vi "Get or Add Sheets.vi"(8 "error in":errorcluster, 11 "SpreadsheetDoc in":refnum<k24>) -> (0 "error out":errorcluster, 2 "Sheets":refnum<k24>, 3 "SpreadsheetDoc out":refnum<k24>)   [LabVIEW 2019, in "Open Xml.lvlib"]
uses:
  Open Xml.lvlib
  D:/git/Open-Xml-LabVIEW/Source/DocumentFormat.OpenXml.dll
  DocumentFormat.OpenXml.dll
  D:/git/Open-Xml-LabVIEW/Source/DocumentFormat.OpenXml.Framework.dll
  DocumentFormat.OpenXml.Framework.dll
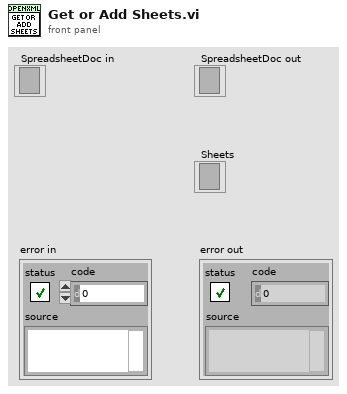
[diagram p1: front panel]
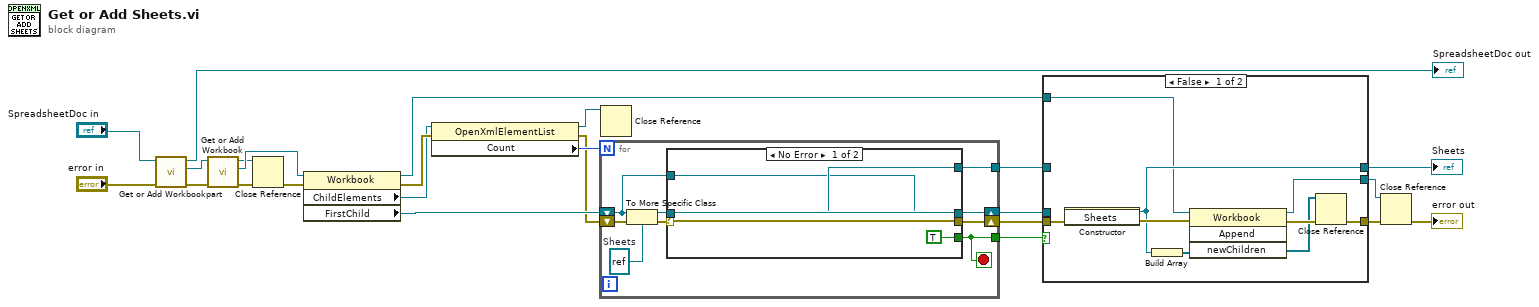
[diagram p0: block diagram]
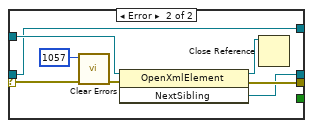
[diagram p2: hidden frame]
diagram:
  n1 = call "Get or Add Workbookpart.vi"("error in"="error in", "SpreadsheetDoc in"="SpreadsheetDoc in") -> ("error out"=w7:errorcluster, "WorkbookPart"=w5:refnum<k24>, "SpreadsheetDoc out"=→"SpreadsheetDoc out":refnum<k24>)  [unwired: 7 in]
  n2 = call "Get or Add Workbook.vi"("error in"=w7, "Workbookpart in"=w5) -> ("error out"=w6:errorcluster, "Workbook"=w4:refnum<k24>, "Workbookpart out"=w2:refnum<k24>)  [unwired: 7 in]
  n3 = Close Reference(reference=w2, error in (no error)=w6) -> (error out=w3:errorcluster)
  n4 = property class="Workbook"(reference=w4, error in=w3) -> (reference out=w11:refnum<k24>, error out=w21:errorcluster, "ChildElements"=w19:refnum<k24>, "FirstChild"=w18:refnum<k24>)
  n5 = property class="OpenXmlElementList"(reference=w19, error in=w21) -> (reference out=w8:refnum<k24>, error out=w17:errorcluster, "Count"=w20:i32)
  n6 = for {
    N: w20 -> [_]
    shift-right: [w28] -> _
    shift-left: w18 -> [w25]
    tunnel: [w26] -> w13
    shift-right: [w27] -> w15
    shift-left: w17 -> [w31]
    tunnel: [w24] -> w1
    stop <- w24 stop-if-true
    w32 = refnum<k24> refnum  # Sheets
    n7 = To More Specific Class(target class=w32, reference=w25, error in=w31) -> (specific class reference=w29:refnum<k24>, error out=w30:errorcluster)
    n8 = case shown="No Error" w30 {
      selector: w30 -> [w33 w44]
      tunnel: w29 -> [w35 w37]
      tunnel: [w34 w41] -> w28
      tunnel: [TRUE _] -> w24
      tunnel: [w33 w42] -> w27
      tunnel: [w35 w37] -> w26
      tunnel: w25 -> [w34 w38]
      frame No Error {
      }
      frame Error {
        n9 = call <vilib>:"Clear Errors.vi"("error in (no error)"=w44, "specific error code to clear (0: all)"=1057) -> ("error out"=w40:errorcluster)  [unwired: 4 in, 1 out]
        n10 = invoke class="OpenXmlElement" method="NextSibling"(reference=w38, error in=w40) -> (reference out=w43:refnum<k24>, error out=w42:errorcluster, "NextSibling"=w41:refnum<k24>)  [unwired: 1 in]
        n11 = Close Reference(reference=w43) -> ()  [unwired: 1 in, 1 out]
      }
    }
  }
  n12 = Close Reference(reference=w8) -> ()  [unwired: 1 in, 1 out]
  n13 = case shown="False" w1 {
    tunnel: w11 -> [_ _]
    tunnel: w15 -> [w52 w56]
    tunnel: [w47 w56] -> w14
    tunnel: w13 -> [_ w55]
    tunnel: [w49 w55] -> w12
    tunnel: w11 -> [w46 w54]
    tunnel: [w45 w54] -> w9
    frame False {
      n14 = constructor class="Sheets"(error in=w52) -> (reference out=w49:refnum<k24>, error out=w51:errorcluster)  [unwired: 2 in, 1 out]
      n15 = Build Array(w49) -> (w48:refnum<k24>[])
      n16 = invoke class="Workbook" method="Append"(reference=w46, error in=w51, "newChildren"=w48) -> (reference out=w45:refnum<k24>, error out=w53:errorcluster, "newChildren"=w50:refnum<k24>[])  [unwired: 1 in, 1 out]
      n17 = Close Reference(reference=w50, error in (no error)=w53) -> (error out=w47:errorcluster)
    }
    frame True {
    }
  }
  "Sheets" <- w12
  n18 = Close Reference(reference=w9, error in (no error)=w14) -> (error out=→"error out":errorcluster)
